vi "niScope Get Virtual Channels Status.vi"(8 "error in":errorcluster, 11 "niScope in":T1={"channel cfg"=[], "sessions"=[], "multi cards"=FALSE, "channels"=0, "type"=enum."n/a", "memory [B/chn]"=0, "ext. clock [Hz]"=0.0, "samples count"=0, "use streaming"=FALSE, "proc setup"={"packet size [smpl]"=0, "current timeout [s]"=0.0, "blk2blk timeout [s]"=0.0, "event time"=timestamp(0 s since 1904-01-01), "temp sampl T [s]"=0.0, "data queue"=refnum, "stop notifier"=refnum, "proc ref"=refnum}, "sample width [B]"=0, "ranges [V]"=[], "trigger setup"={"coupling"=1, "level [V]"=0.0, "slope"=0, "mode"=enum."Immediate"}, "fs [Hz]"=0.0, "bitres [bit]"=0, "clock source"=enum."VAL_NO_SOURCE"} {"trigger setup"."level [V]" format="%.2f"; "trigger setup"."coupling" items=["AC"=0, "DC"=1, "HF Reject"=3, "LF Reject"=4, "AC Plus HF Reject"=1001]; "channel cfg"."Range [Vpk]" min=0.0; "channel cfg"."Channel" min=0}) -> (0 "error out":errorcluster, 1 "points done":i64[](array[numeric]), 2 "temperatures [deg C]":dbl[](array[numeric]), 3 "niScope out":T1={"channel cfg"=[], "sessions"=[], "multi cards"=FALSE, "channels"=0, "type"=enum."n/a", "memory [B/chn]"=0, "ext. clock [Hz]"=0.0, "samples count"=0, "use streaming"=FALSE, "proc setup"={"packet size [smpl]"=0, "current timeout [s]"=0.0, "blk2blk timeout [s]"=0.0, "event time"=timestamp(0 s since 1904-01-01), "temp sampl T [s]"=0.0, "data queue"=refnum, "stop notifier"=refnum, "proc ref"=refnum}, "sample width [B]"=0, "ranges [V]"=[], "trigger setup"={"coupling"=1, "level [V]"=0.0, "slope"=0, "mode"=enum."Immediate"}, "fs [Hz]"=0.0, "bitres [bit]"=0, "clock source"=enum."VAL_NO_SOURCE"} {"trigger setup"."level [V]" format="%.2f"; "trigger setup"."coupling" items=["AC"=0, "DC"=1, "HF Reject"=3, "LF Reject"=4, "AC Plus HF Reject"=1001]; "channel cfg"."Range [Vpk]" min=0.0; "channel cfg"."Channel" min=0}, 4 "all channels sampling?":bool)   [LabVIEW 2020, in "niScope Virtual Digitizer.lvlib"]
doc: "Reads status of cards designated by virtual channels in the session. Returns array of temperatures and 'points done', one item for each virtual channel."
uses:
  niScope Virtual Digitizer.lvlib
  niScope Session.ctl
  niScope Virtual Channel Config.ctl
  niScope Virtual Channel Mode.ctl
  niScope Virtual Channel Input Z.ctl
  niScope Virtual Channel Coupling.ctl
  niScope Type.ctl
  niScope Digitizing Process Options.ctl
  niScope Data Packet.ctl
  niScope Trigger Setup.ctl
  <instrlib>/niScope/Controls/niScope trigger coupling.ctl
  <instrlib>/niScope/Controls/niScope trigger slope.ctl
  niScope Reference Clock.ctl
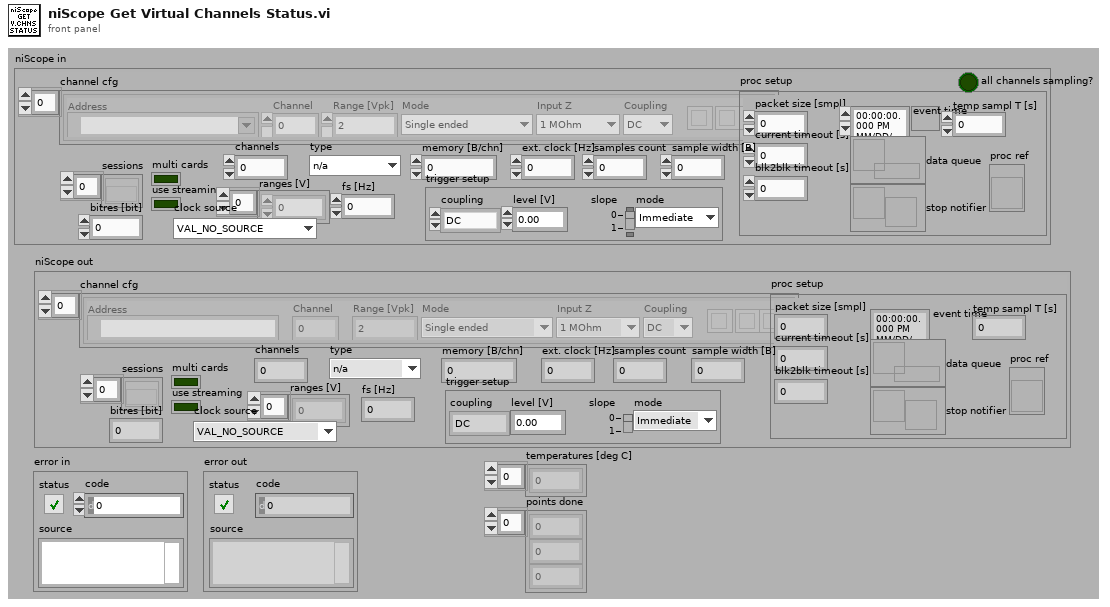
[diagram p1: front panel]
types:
  T1 = typedef "niScope Virtual Digitizer.lvlib/niScope Session.ctl" = cluster{"channel cfg":T2[], "sessions":refnum<k20>[], "multi cards":bool, "channels":i32, "type":T6, "memory [B/chn]":i32, "ext. clock [Hz]":dbl, "samples count":i64, "use streaming":bool, "proc setup":T7, "sample width [B]":i32, "ranges [V]":dbl[], "trigger setup":T8, "fs [Hz]":dbl, "bitres [bit]":i32, "clock source":T11}
  T2 = typedef "niScope Virtual Digitizer.lvlib/niScope Virtual Channel Config.ctl" = cluster{"Address":refnum<k15>, "Channel":i32, "Mode":T3, "Input Z":T4, "Coupling":T5, "Range [Vpk]":dbl, "btn clr":bool, "btn up":bool, "btn down":bool}
  T3 = typedef "niScope Virtual Digitizer.lvlib/niScope Virtual Channel Mode.ctl" = enum16{"Single ended", "Unbal. differential", "Differential"}
  T4 = typedef "niScope Virtual Digitizer.lvlib/niScope Virtual Channel Input Z.ctl" = enum16{"1 MOhm", "50 Ohm"}
  T5 = typedef "niScope Virtual Digitizer.lvlib/niScope Virtual Channel Coupling.ctl" = enum16{"AC", "DC", "GND"}
  T6 = typedef "niScope Virtual Digitizer.lvlib/niScope Type.ctl" = enum16{"n/a", "5922"}
  T7 = typedef "niScope Virtual Digitizer.lvlib/niScope Digitizing Process Options.ctl" = cluster{"packet size [smpl]":i64, "current timeout [s]":dbl, "blk2blk timeout [s]":dbl, "event time":timestamp, "temp sampl T [s]":dbl, "data queue":refnum<queue>, "stop notifier":refnum<notifier>, "proc ref":refnum<vi>}
  T8 = typedef "niScope Virtual Digitizer.lvlib/niScope Trigger Setup.ctl" = cluster{"coupling":T9, "level [V]":dbl, "slope":T10, "mode":enum16{"Immediate", "External", "Level"}}
  T9 = typedef "niScope trigger coupling.ctl" = u16
  T10 = typedef "niScope trigger slope.ctl" = i32
  T11 = typedef "niScope Virtual Digitizer.lvlib/niScope Reference Clock.ctl" = enum16{"VAL_NO_SOURCE", "VAL_CLK_IN", "VAL_PXI_CLOCK", "VAL_EXTERNAL"}
  T12 = typedef "niScope Virtual Digitizer.lvlib/niScope Physical Cards.ctl" = cluster{"chn lst":i32[], "addr":refnum<k15>, "chn pos":i32[]}
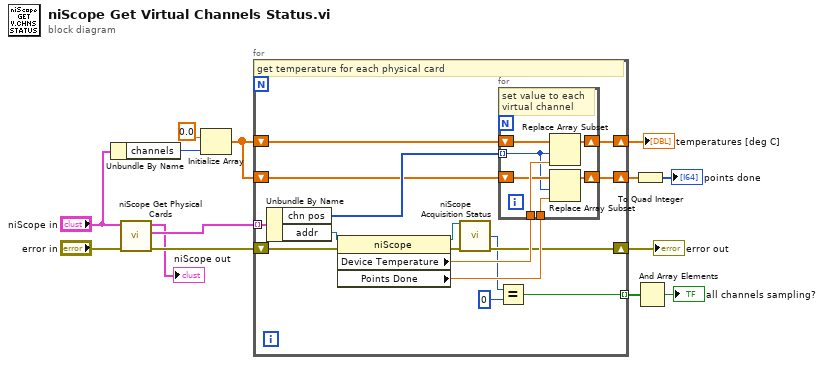
[diagram p0: block diagram]
diagram:
  n1 = Unbundle By Name("niScope in") -> ("channels"=w6:i32)
  n2 = call "niScope Get Physical Cards.vi"("error in"="error in", "niScope in"="niScope in") -> ("error out"=w12:errorcluster, "card list"=w13:T12[], "niScope out"=→"niScope out":T1)  [unwired: 7 in]
  n3 = Initialize Array(0.0, w6) -> (w5:dbl[])
  n4 = for {
    tunnel: w13 -> [w30] mode=indexing
    shift-right: [w19] -> w8
    shift-left: w12 -> [w28]
    shift-right: [w27] -> w7
    shift-left: w5 -> [w26]
    shift-right: [w23] -> w4
    shift-left: w5 -> [w22]
    tunnel: [w15] -> w2 mode=indexing
    # "get temperature for each physical card"
    n5 = Unbundle By Name(w30) -> ("chn pos"=w25:i32[], "addr"=w29:refnum<k15>)
    n6 = property class="niScope"(reference=w29, error in=w28) -> (reference out=w18:refnum<k15>, error out=w20:errorcluster, "Device Temperature"=w24:dbl, "Points Done"=w21:dbl)
    n7 = call <instrlib>:"niScope Acquisition Status.vi"("instrument handle"=w18, "error in"=w20) -> ("acquisition status"=w17:i32, "error out"=w19:errorcluster)  [unwired: 11 in, 1 out]
    n8 = Equal?(x=w17, y=0) -> (x = y?=w15:bool)
    n9 = for {
      tunnel: w25 -> [w31] mode=indexing
      tunnel: w24 -> [w35]
      tunnel: w21 -> [w32]
      shift-right: [w37] -> w27
      shift-left: w26 -> [w36]
      shift-right: [w34] -> w23
      shift-left: w22 -> [w33]
      # "set value to each\nvirtual channel"
      n10 = Replace Array Subset(array=w36, new element=w35, index=w31) -> (w37:dbl[])
      n11 = Replace Array Subset(array=w33, new element=w32, index=w31) -> (w34:dbl[])
    }
  }
  "error out" <- w8
  "temperatures [deg C]" <- w7
  n12 = To Quad Integer(1:w4) -> (0:→"points done":i64[])
  n13 = And Array Elements(Boolean array=w2) -> (logical AND=→"all channels sampling?":bool)
